vi "Using_Array_Over_Threshold.vi"() -> ()   [LabVIEW 2020]
panel:
  out "OUTPUT ARRAY":dbl[](array[numeric]) format="%#_3g"
  out "numbers (0 to 1)":dbl[](array[numeric]) format="%#_3g"
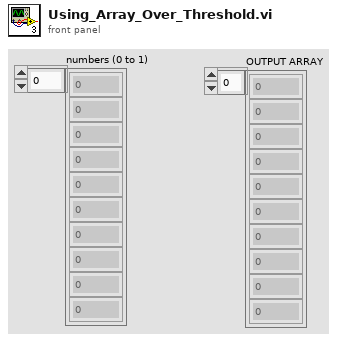
[diagram p1: front panel]
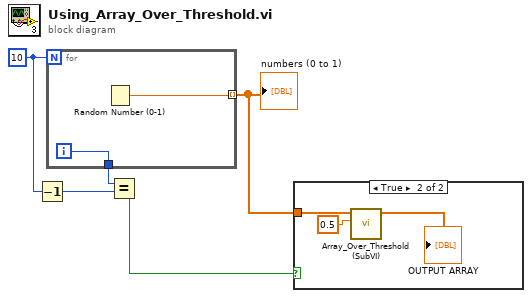
[diagram p0: block diagram]
diagram:
  w5 = 10
  n1 = Decrement(x=w5) -> (x-1=w4:i32)
  n2 = for {
    N: w5 -> [_]
    tunnel: [w7] -> w1 mode=indexing
    tunnel: [w6] -> w3
    i -> [w6]
    n3 = Random Number (0-1)() -> (number: 0 to 1=w7:dbl)
  }
  "numbers (0 to 1)" <- w1
  n4 = Equal?(x=w3, y=w4) -> (x = y?=w2:bool)
  n5 = case shown="True" w2 {
    tunnel: w1 -> [_ w10]
    frame False {
    }
    frame True {
      n6 = call "Array_Over_Threshold (SubVI).vi"("Threshold"=0.5, "Start Array"=w10) -> ("Array"=→"OUTPUT ARRAY":dbl[])  [unwired: 9 in]
    }
  }
